vi "RW Rect ROI.vi"(7 "Read/Write":enum16{"Read", "Write"}(ring), 8 "error in (no error)":errorcluster, 9 "directory Path":string="Ini\\ROI.ini", 10 "section":string, 11 "ROI Descriptor":T1 {"Contours"."Type" items=["No Selection", "Point", "Line", "Rectangle", "Oval", "Polygon", "Freehand Region", "Annulus", "Unused2", "Unused3", "Broken Line", "Freehand Line", "Rotated Rectangle"]}) -> (0 "error out":errorcluster, 3 "ROI Descriptor Out":T1 {"Contours"."Type" items=["No Selection", "Point", "Line", "Rectangle", "Oval", "Polygon", "Freehand Region", "Annulus", "Unused2", "Unused3", "Broken Line", "Freehand Line", "Rotated Rectangle"]})   [LabVIEW 2017]
uses:
  Beta/File/Control/Parent path.ctl
  <vilib>/Utility/config.llb/Write Key (I32).vi
  <vilib>/Utility/config.llb/Write Key (Double).vi
  <vilib>/Utility/config.llb/Read Key (I32).vi
  <vilib>/Utility/config.llb/Read Key (Double).vi
  Beta/File/File.lvlib
  <vilib>/Utility/config.llb/NI_LVConfig.lvlib
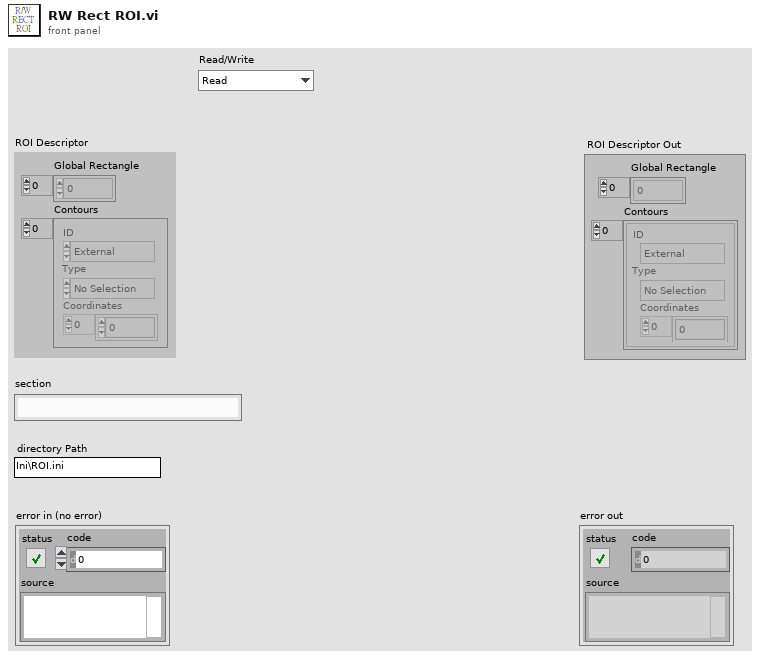
[diagram p1: front panel]
types:
  T1 = typedef "ROI Descriptor" = cluster{"Global Rectangle":i32[], "Contours":cluster{"ID":enum32{"External", "Internal"}, "Type":u32, "Coordinates":i32[]}[]}
  T2 = typedef "File.lvlib/Parent path.ctl" = enum16{"Project", "Data", "Log"}
  T3 = typedef "IMAQ Rectangle" = cluster{"Left":i32, "Top":i32, "Right":i32, "Bottom":i32, "Rotation":dbl}
  T4 = typedef "NI_LVConfig.lvlib/Config Data RefNum.ctl" = refnum<k1>
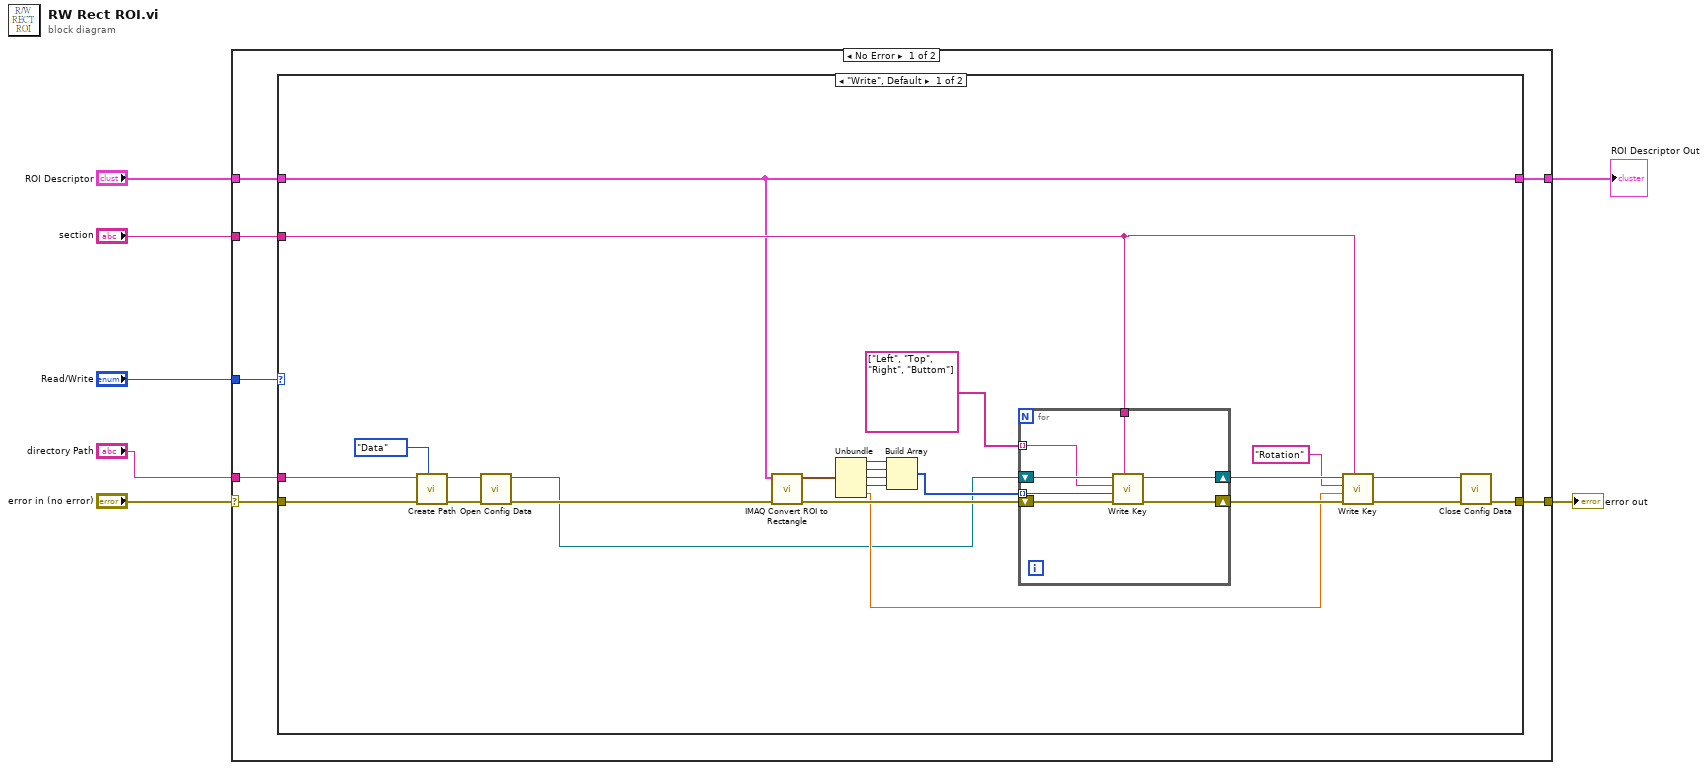
[diagram p0: block diagram]
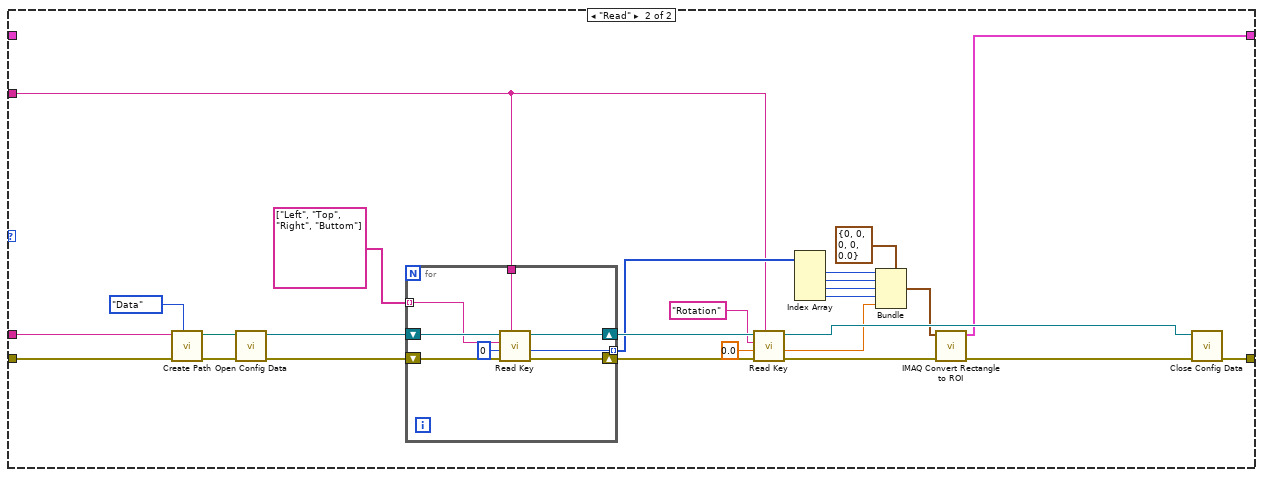
[diagram p2: hidden frame]
diagram:
  n1 = case shown="No Error" "error in (no error)" {
    selector: "error in (no error)" -> [w14 w81]
    tunnel: [w13 w81] -> w6
    tunnel: "Read/Write" -> [w12 _]
    tunnel: "section" -> [w11 _]
    tunnel: "directory Path" -> [w10 _]
    tunnel: "ROI Descriptor" -> [w9 w80]
    tunnel: [w8 w80] -> w1
    frame No Error {
      n2 = case shown="\"Write\", Default" w12 {
        tunnel: w14 -> [w38 w71]
        tunnel: [w32 w65] -> w13
        tunnel: w11 -> [w19 w51]
        tunnel: w10 -> [w18 w46]
        tunnel: w9 -> [w15 _]
        tunnel: [w15 w47] -> w8
        frame "Write", Default {
          n3 = call "Create Path.vi"("Parent path"=Parent_path."Data", "error in (no error)"=w38, "Directory"=w18) -> ("error out"=w36:errorcluster, "Path"=w35:path)  [unwired: 7 in]
          n4 = call <vilib>:"Open Config Data.vi"("error in (no error)"=w36, "configuration file path"=w35) -> ("error out"=w34:errorcluster, "refnum"=w20:T4)  [unwired: 7 in, 1 out]
          n5 = call "IMAQ Convert ROI to Rectangle"("error in (no error)"=w34, "ROI Descriptor"=w15) -> ("error out"=w28:errorcluster, "Rectangle"=w27:T3)  [unwired: 7 in]
          n6 = Unbundle(w27) -> ("Left"=w25:i32, "Top"=w24:i32, "Right"=w23:i32, "Bottom"=w22:i32, "Rotation"=w26:dbl)
          n7 = Build Array(w25, w24, w23, w22) -> (w21:i32[])
          n8 = for {
            shift-right: [w43] -> w30
            shift-left: w20 -> [w45]
            shift-right: [w42] -> w29
            shift-left: w28 -> [w44]
            tunnel: string[] ["Left", "Top", "Right", "Buttom"] ("Rect") -> [w41] mode=indexing
            tunnel: w19 -> [w40]
            tunnel: w21 -> [w39] mode=indexing
            n9 = call-poly <vilib>:"Write Key.vi"("section"=w40, "error in (no error)"=w44, "value"=w39, "key"=w41, "refnum"=w45) -> ("error out"=w42:errorcluster, "refnum out"=w43:T4)  [unwired: 4 in, 1 out]
          }
          n10 = call-poly <vilib>:"Write Key.vi"("section"=w19, "error in (no error)"=w29, "value"=w26, "key"="Rotation" ("Angel"), "refnum"=w30) -> ("error out"=w33:errorcluster, "refnum out"=w31:T4)  [unwired: 4 in, 1 out]
          n11 = call <vilib>:"Close Config Data.vi"("error in (no error)"=w33, "refnum"=w31) -> ("error out"=w32:errorcluster)  [unwired: 8 in, 1 out]
        }
        frame "Read" {
          n12 = call "Create Path.vi"("Parent path"=Parent_path."Data", "error in (no error)"=w71, "Directory"=w46) -> ("error out"=w69:errorcluster, "Path"=w68:path)  [unwired: 7 in]
          n13 = call <vilib>:"Open Config Data.vi"("error in (no error)"=w69, "configuration file path"=w68) -> ("error out"=w66:errorcluster, "refnum"=w67:T4)  [unwired: 7 in, 1 out]
          n14 = for {
            shift-right: [w77] -> w63
            shift-left: w67 -> [w79]
            shift-right: [w76] -> w62
            shift-left: w66 -> [w78]
            tunnel: [w75] -> w60 mode=indexing
            tunnel: string[] ["Left", "Top", "Right", "Buttom"] ("Rect") -> [w74] mode=indexing
            tunnel: w51 -> [w73]
            n15 = call-poly <vilib>:"Read Key.vi"("section"=w73, "error in (no error)"=w78, "default value"=0, "key"=w74, "refnum"=w79) -> ("error out"=w76:errorcluster, "value"=w75:i32, "refnum out"=w77:T4)  [unwired: 3 in, 1 out]
          }
          n16 = call-poly <vilib>:"Read Key.vi"("section"=w51, "error in (no error)"=w62, "default value"=0.0, "key"="Rotation" ("Angel"), "refnum"=w63) -> ("error out"=w61:errorcluster, "value"=w54:dbl, "refnum out"=w64:T4)  [unwired: 3 in, 1 out]
          n17 = Index Array(array=w60) -> (element #1=w58:i32, element #2=w57:i32, element #3=w56:i32, element #4=w55:i32)  [unwired: 4 in]
          n18 = Bundle(cluster=T3 {"Left"=0, "Top"=0, "Right"=0, "Bottom"=0, "Rotation"=0.0} ("Rectangle"), "Left"=w58, "Top"=w57, "Right"=w56, "Bottom"=w55, "Rotation"=w54) -> (w53:T3)
          n19 = call "IMAQ Convert Rectangle to ROI"("error in (no error)"=w61, "Rectangle"=w53) -> ("error out"=w48:errorcluster, "ROI Descriptor"=w47:T1)  [unwired: 7 in]
          n20 = call <vilib>:"Close Config Data.vi"("error in (no error)"=w48, "refnum"=w64) -> ("error out"=w65:errorcluster)  [unwired: 8 in, 1 out]
        }
      }
    }
    frame Error {
    }
  }
  "error out" <- w6
  "ROI Descriptor Out" <- w1
